vi "Parse DB TX Labels.vi"(8 "error in":errorcluster, 9 "acyclic transfer count":u32, 10 "scheduled transfer count":u32, 11 "Channel Config":u32) -> (0 "error out":errorcluster, 2 "Labels":T1[](array[typedef]) {"scheduleBuildUnit" items=["Millisecond", "Microsecond"]})   [LabVIEW 2016]
uses:
  Controls/AIT_Label.ctl
  Controls/AIT_Word.ctl
  Controls/ARINCParam.ctl
  Shared/Controls and Global/TransferType.ctl
  Ballard Arinc-429 System Explorer.lvlib
  <userlib>/ARINC-429/Owl429.lvlib
  Shared/Ballard Arinc-429 Shared.lvlib
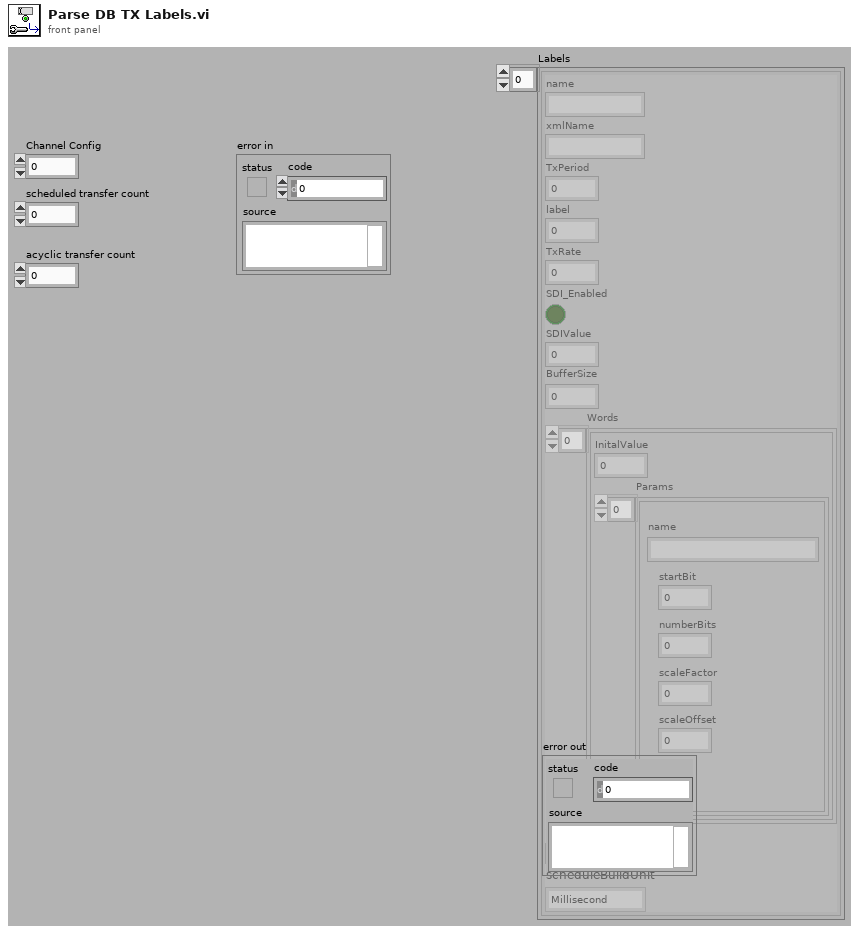
[diagram p1: front panel]
types:
  T1 = typedef "Ballard Arinc-429 System Explorer.lvlib/AIT_Label.ctl" = cluster{"name":string, "xmlName":string, "TxPeriod":u32, "label":u32, "TxRate":dbl, "SDI_Enabled":bool, "SDIValue":u8, "BufferSize":u32, "Words":T2[], "TransferType":T4, "scheduleBuildUnit":i32}
  T2 = typedef "Ballard Arinc-429 System Explorer.lvlib/AIT_Word.ctl" = cluster{"InitalValue":u32, "Params":T3[]}
  T3 = typedef "Ballard Arinc-429 System Explorer.lvlib/ARINCParam.ctl" = cluster{"name":string, "startBit":i32, "numberBits":i32, "scaleFactor":dbl, "scaleOffset":dbl, "signed":bool}
  T4 = typedef "Ballard Arinc-429 Shared.lvlib/TransferType.ctl" = enum16{"ScheduledLabel", "Acyclic", "Block", "Strobe"}
  T5 = typedef "Owl429.lvlib/Owl429TxLabelConfigType.ctl" = enum16{"OWL429_BLOCK_TRANSFER_CONFIG", "OWL429_SCHEDULED_LABEL_CONFIG", "OWL429_STROBE_TRANSFER_CONFIG"}
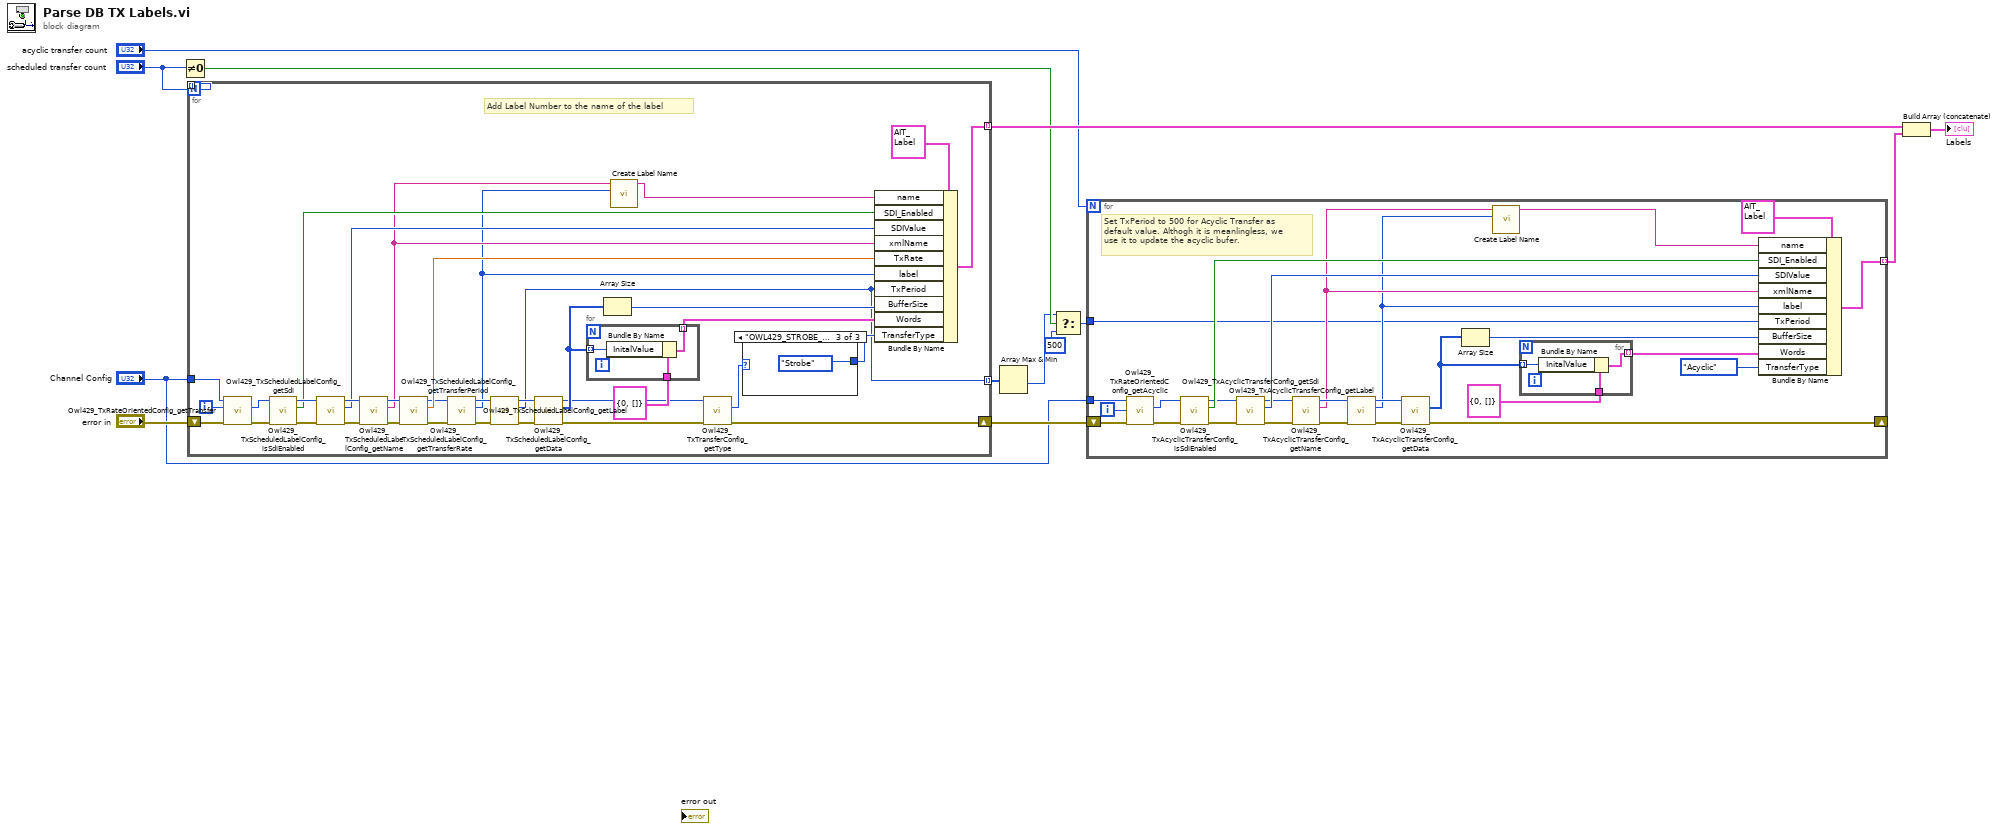
[diagram p0: block diagram]
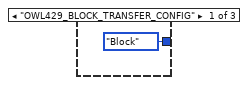
[diagram p2: hidden frame]
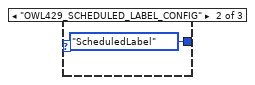
[diagram p3: hidden frame]
diagram:
  n1 = Not Equal To 0?(x="scheduled transfer count") -> (x != 0?=w4:bool)
  n2 = for {
    N: "scheduled transfer count" -> [w14]
    shift-right: [w20] -> w9
    shift-left: "error in" -> [w49]
    tunnel: "Channel Config" -> [w48]
    tunnel: [w46] -> w13 mode=indexing
    tunnel: [w15] -> w6 mode=indexing
    tunnel: [w14] -> _ mode=indexing
    i -> [w47]
    # "Add Label Number to the name of the label"
    n3 = call <userlib>:"Owl429_TxRateOrientedConfig_getTransfer.vi"("error in (no error)"=w49, "transfer handle"=w47, "config handle"=w48) -> ("error out"=w36:errorcluster, "transfer config handle"=w22:u64)  [unwired: 6 in, 1 out]
    n4 = call <userlib>:"Owl429_TxScheduledLabelConfig_isSdiEnabled.vi"("error in (no error)"=w36, "label config handle"=w22) -> ("error out"=w34:errorcluster, "sdi enabled"=w31:bool, "label config handle"=w33:u64)  [unwired: 7 in]
    n5 = call <userlib>:"Owl429_TxScheduledLabelConfig_getSdi.vi"("error in (no error)"=w34, "label config handle"=w33) -> ("error out"=w32:errorcluster, "sdi"=w30:u8, "label config handle"=w35:u64)  [unwired: 7 in]
    n6 = call <userlib>:"Owl429_TxScheduledLabelConfig_getName.vi"("error in (no error)"=w32, "label config handle"=w35) -> ("error out"=w37:errorcluster, "label"=w29:string, "label config handle"=w38:u64)  [unwired: 7 in]
    n7 = call <userlib>:"Owl429_TxScheduledLabelConfig_getTransferRate.vi"("error in (no error)"=w37, "label config handle"=w38) -> ("error out"=w42:errorcluster, "transfer rate"=w45:dbl, "label config handle"=w43:u64)  [unwired: 7 in]
    n8 = call <userlib>:"Owl429_TxScheduledLabelConfig_getLabel.vi"("error in (no error)"=w42, "label config handle"=w43) -> ("error out"=w44:errorcluster, "label"=w27:u8, "label config handle"=w41:u64)  [unwired: 7 in]
    n9 = call <userlib>:"Owl429_TxScheduledLabelConfig_getTransferPeriod.vi"("error in (no error)"=w44, "label config handle"=w41) -> ("error out"=w40:errorcluster, "transfer period"=w15:u32, "label config handle"=w39:u64)  [unwired: 7 in]
    n10 = call <userlib>:"Owl429_TxScheduledLabelConfig_getData.vi"("error in (no error)"=w40, "scheduled label config handle"=w39) -> ("error out"=w21:errorcluster, "data buffer"=w25:u32[], "scheduled label config handle"=w19:u64)  [unwired: 7 in]
    n11 = for {
      tunnel: w25 -> [w55] mode=indexing
      tunnel: T2 {"InitalValue"=0, "Params"=[]} ("Word") -> [w54]
      tunnel: [w53] -> w23 mode=indexing
      n12 = Bundle By Name(cluster=w54, "InitalValue"=w55) -> (w53:T2)
    }
    n13 = Array Size(array=w25) -> (size(s)=w26:i32)
    n14 = call "Create Label Name.vi"("label number"=w27, "label XML name"=w29) -> ("label name"=w28:string)  [unwired: 9 in]
    n15 = call <userlib>:"Owl429_TxTransferConfig_getType.vi"("error in (no error)"=w21, "transfer config handle"=w19) -> ("error out"=w20:errorcluster, "label config type"=w18:T5)  [unwired: 7 in, 1 out]
    n16 = case shown="\"OWL429_STROBE_TRANSFER_CONFIG\", Default" w18 {
      tunnel: [TransferType."Block" ("TransferType") TransferType."ScheduledLabel" ("TransferType") TransferType."Strobe" ("TransferType")] -> w17
      frame "OWL429_BLOCK_TRANSFER_CONFIG" {
      }
      frame "OWL429_SCHEDULED_LABEL_CONFIG" {
      }
      frame "OWL429_STROBE_TRANSFER_CONFIG", Default {
      }
    }
    n17 = Bundle By Name(cluster=T1 {"name"="", "xmlName"="", "TxPeriod"=0, "label"=0, "TxRate"=0.0, "SDI_Enabled"=FALSE, "SDIValue"=0, "BufferSize"=0, "Words"=[], "TransferType"=enum."ScheduledLabel", "scheduleBuildUnit"=0} ("Label"), "name"=w28, "SDI_Enabled"=w31, "SDIValue"=w30, "xmlName"=w29, "TxRate"=w45, "label"=w27, "TxPeriod"=w15, "BufferSize"=w26, "Words"=w23, "TransferType"=w17) -> (w46:T1)
  }
  n18 = Array Max & Min(array=w6) -> (min value=w3:u32)  [unwired: 3 out]
  n19 = Select(t=w3, s=w4, f=u32 500) -> (s? t:f=w1:u32)
  n20 = for {
    N: "acyclic transfer count" -> [_]
    shift-right: [w63] -> _
    shift-left: w9 -> [w82]
    tunnel: "Channel Config" -> [w81]
    tunnel: [w76] -> w7 mode=indexing
    tunnel: w1 -> [w56]
    i -> [w80]
    # "Set TxPeriod to 500 for Acyclic Transfer as\ndefault value. Althogh it is meanlingless, we\nuse it to update the acyclic bufer."
    n21 = call <userlib>:"Owl429_TxRateOrientedConfig_getAcyclic.vi"("error in (no error)"=w82, "acyclic handle"=w80, "config handle"=w81) -> ("error out"=w75:errorcluster, "acyclic config handle"=w71:u64)  [unwired: 6 in, 1 out]
    n22 = call "Owl429_TxAcyclicTransferConfig_isSdiEnabled.vi"("error in (no error)"=w75, "acyclic config handle"=w71) -> ("error out"=w74:errorcluster, "sdi enabled"=w70:bool, "acyclic config handle"=w68:u32)  [unwired: 7 in]
    n23 = call "Owl429_TxAcyclicTransferConfig_getSdi.vi"("error in (no error)"=w74, "acyclic config handle"=w68) -> ("error out"=w73:errorcluster, "sdi"=w69:u8, "acyclic config handle"=w67:u32)  [unwired: 7 in]
    n24 = call "Owl429_TxAcyclicTransferConfig_getName.vi"("error in (no error)"=w73, "acyclic config handle"=w67) -> ("error out"=w72:errorcluster, "label"=w65:string, "acyclic config handle"=w66:u32)  [unwired: 7 in]
    n25 = call "Owl429_TxAcyclicTransferConfig_getLabel.vi"("error in (no error)"=w72, "acyclic config handle"=w66) -> ("error out"=w60:errorcluster, "label"=w57:u8, "acyclic config handle"=w61:u32)  [unwired: 7 in]
    n26 = call <userlib>:"Owl429_TxAcyclicTransferConfig_getData.vi"("error in (no error)"=w60, "acyclic config handle"=w61) -> ("error out"=w63:errorcluster, "data buffer"=w58:u32[])  [unwired: 7 in, 1 out]
    n27 = Array Size(array=w58) -> (size(s)=w59:i32)
    n28 = call "Create Label Name.vi"("label number"=w57, "label XML name"=w65) -> ("label name"=w78:string)  [unwired: 9 in]
    n29 = for {
      tunnel: w58 -> [w85] mode=indexing
      tunnel: T2 {"InitalValue"=0, "Params"=[]} ("Word") -> [w84]
      tunnel: [w83] -> w62 mode=indexing
      n30 = Bundle By Name(cluster=w84, "InitalValue"=w85) -> (w83:T2)
    }
    n31 = Bundle By Name(cluster=T1 {"name"="", "xmlName"="", "TxPeriod"=0, "label"=0, "TxRate"=0.0, "SDI_Enabled"=FALSE, "SDIValue"=0, "BufferSize"=0, "Words"=[], "TransferType"=enum."ScheduledLabel", "scheduleBuildUnit"=0} ("Label"), "name"=w78, "SDI_Enabled"=w70, "SDIValue"=w69, "xmlName"=w65, "label"=w57, "TxPeriod"=w56, "BufferSize"=w59, "Words"=w62, "TransferType"=TransferType."Acyclic") -> (w76:T1)
  }
  n32 = Build Array (concatenate)(w13, w7) -> (→"Labels":T1[])
